vi "Lab Panel V5.25.vi"() -> ()   [LabVIEW 2017] (continued)
                                n852 = Bundle(cluster=w1518, "TL"=w1516, "TN"=w1516) -> (w1517:cluster{"TL":dbl, "TN":dbl})
                                n853 = local write "TEMP START LAB03-2"(w1517) -> ()
                              }
                            }
                          }
                        }
                      }
                    }
                  }
                }
              }
              event "RUN LAB04-1": Value Change {
                n854 = event-data() -> ("NewVal"=w1523:bool)  [unwired: 1 in, 5 out]
                n855 = local write "run lab04-1"(w1523) -> ()
                n856 = case shown="True" w1523 {
                  tunnel: w1529 -> [_ w1567]
                  tunnel: w1528 -> [_ w1566]
                  tunnel: w1526 -> [w1531 w1565]
                  tunnel: w1527 -> [_ w1564]
                  tunnel: w1525 -> [_ w1563]
                  tunnel: [w1530 w1562] -> w1524
                  tunnel: w1522 -> [_ w1561]
                  tunnel: w1521 -> [_ w1560]
                  tunnel: w1520 -> [_ w1559]
                  tunnel: w1519 -> [_ w1557]
                  frame False {
                    # "stop test"
                    n857 = stacked-sequence {
                      tunnel: w1531 -> [w1540 _]
                      tunnel: [w1532 _] -> w1530
                      frame #0 {
                        n858 = local read "DISP LAB04-1"() -> (w1539:T4)
                        n859 = Unbundle(w1539) -> ("CYCLE"=w1537:dbl, "MINS"=w1538:dbl)  [unwired: 1 out]
                        n860 = case shown="\"CYCLE TEST\"" w1540 {
                          tunnel: w1538 -> [_ _ w1547]
                          tunnel: w1537 -> [w1545 w1546 _]
                          tunnel: [w1545 w1546 w1547] -> w1536
                          frame "CHART TEST", Default {
                          }
                          frame "CYCLE TEST" {
                          }
                          frame "T-RISE TEST" {
                          }
                        }
                        n861 = local read "TDMS LAB04-1"() -> (w1544:refnum<k34>)
                        n862 = Build Array("STOPPED") -> (w1541:string[])
                        n863 = Build Array(w1536) -> (w1535:dbl[])
                        n864 = TDMS Write(0:w1544, 5:"TEST RESULT", 7:w1541, 9:w1535) -> (4:w1533:refnum<k34>, 15:w1534:errorcluster)  [unwired: 2 in, 2 out]
                        n865 = TDMS Close(8:w1534, 11:w1533) -> (0:w1532:errorcluster)  [unwired: 1 out]
                      }
                      frame #1 {
                        n866 = local read "DISP LAB04-1"() -> (w1551:T4)
                        n867 = stacked-sequence {
                          tunnel: "LAB04-1" -> [w1553 w1555]
                          frame #0 {
                            n868 = call "sub vi - defrag tdms v1.vi"("panel id"=w1553) -> ("error out"=w1552:errorcluster)  [unwired: 10 in]
                            n869 = local write "data file error"(w1552) -> ()
                          }
                          frame #1 {
                            n870 = call "Save data file (stop) v3.vi"("panel id"=w1555) -> ("network file save error"=w1554:errorcluster)  [unwired: 9 in, 1 out]
                            n871 = local write "RESULT LAB04-1"(FALSE) -> ()
                            n872 = local write "data file error"(w1554) -> ()
                          }
                        }
                        n873 = Bundle(cluster=w1551, "STATUS"="STOP") -> (w1549:T4)  [unwired: 2 in]
                        n874 = local write "DISP LAB04-1"(w1549) -> ()
                      }
                    }
                  }
                  frame True {
                    n875 = local read "SIG LAB04-1"() -> (w1558:T2)
                    n876 = stacked-sequence {
                      seq-local: [w1569 _] -> [_ w1573]
                      tunnel: w1567 -> [_ w1583]
                      tunnel: w1566 -> [_ w1582]
                      tunnel: w1565 -> [_ w1581]
                      tunnel: w1564 -> [_ w1580]
                      tunnel: w1563 -> [_ w1579]
                      tunnel: [_ w1578] -> w1562
                      tunnel: w1561 -> [_ w1577]
                      tunnel: w1560 -> [_ w1576]
                      tunnel: w1559 -> [_ w1575]
                      tunnel: w1558 -> [w1568 w1574]
                      tunnel: w1557 -> [_ w1572]
                      frame #0 {
                        n877 = Unbundle(w1568) -> ("AMPS"=w1571:dbl)  [unwired: 4 out]
                        n878 = call "Check For Amps on v1.vi"("ID"="LAB04-1", "amps"=w1571) -> ("amps"=w1569:bool)  [unwired: 9 in]
                      }
                      frame #1 {
                        n879 = case shown="True" w1573 {
                          tunnel: w1583 -> [_ w1596]
                          tunnel: w1582 -> [_ w1595]
                          tunnel: w1581 -> [_ w1594]
                          tunnel: w1580 -> [_ w1593]
                          tunnel: w1579 -> [_ w1592]
                          tunnel: [errorcluster {"status"=FALSE, "code"=0, "source"=""} ("error out") w1591] -> w1578
                          tunnel: w1577 -> [_ w1590]
                          tunnel: w1576 -> [_ w1589]
                          tunnel: w1575 -> [_ w1588]
                          tunnel: w1574 -> [_ w1587]
                          tunnel: w1572 -> [_ w1586]
                          frame False {
                            w1584 = FALSE
                            n880 = local write "RUN LAB04-1"(w1584) -> ()
                            n881 = local write "run lab04-1"(w1584) -> ()
                          }
                          frame True {
                            n882 = stacked-sequence {
                              seq-local: [w1597 _ _ _ _] -> [_ w1621 _ _ _]
                              tunnel: w1596 -> [w1602 _ _ _ _]
                              tunnel: w1595 -> [w1598 _ _ _ _]
                              tunnel: w1594 -> [w1612 _ _ _ _]
                              tunnel: w1593 -> [w1605 _ _ _ _]
                              tunnel: w1592 -> [w1600 _ _ _ _]
                              tunnel: [_ w1616 _ _ _] -> w1591
                              tunnel: w1590 -> [_ _ _ w1642 _]
                              tunnel: w1589 -> [_ _ _ w1641 _]
                              tunnel: w1588 -> [_ _ _ w1640 _]
                              tunnel: w1587 -> [_ _ _ _ _]
                              tunnel: w1586 -> [_ _ _ _ w1656]
                              frame #0 {
                                w1599 = "\\"
                                n883 = local read "SET LAB04-1"() -> (w1607:T5)
                                n884 = case shown="\"CYCLE TEST\"" w1612 {
                                tunnel: ["L04-1-CHART TEST-" "L04-1-CYCLE TEST-" "L04-1-T-RISE TEST-"] -> w1608
                                frame "CHART TEST", Default {
                                }
                                frame "CYCLE TEST" {
                                }
                                frame "T-RISE TEST" {
                                }
                                }
                                n885 = Unbundle(w1607) -> ("DESCRIPTION"=w1606:string)  [unwired: 4 out]
                                n886 = Concatenate Strings(w1602, "\\", w1600, w1599, w1598, w1599) -> (w1609:string)
                                n887 = String To Path(string=w1609) -> (path=w1611:path)
                                n888 = Concatenate Strings(w1609, w1608, w1606, "-", w1605, ".tdms") -> (w1597:string)
                                n889 = Create Folder(path (use dialog)=w1611) -> (error out=w1610:errorcluster)  [unwired: 2 in, 2 out]
                                n890 = global write "Global 1.vi" "LAB04-1 FILE"(w1597) -> ()
                                n891 = call <vilib>:"Clear Errors.vi"("error in (no error)"=w1610) -> ()  [unwired: 5 in, 2 out]
                              }
                              frame #1 {
                                (unwired) FALSE
                                n892 = String To Path(string=w1621) -> (path=w1617:path)
                                n893 = TDMS Open(6:FALSE, 10:T21."create or replace" ("operation (0:open)"), 11:w1617) -> (0:w1616:errorcluster, 3:→"TDMS LAB04-1":refnum<k34>)  [unwired: 4 in]
                              }
                              frame #2 {
                                n894 = local read "SET LAB04-1"() -> (w1627:T5)
                                n895 = local read "TDMS LAB04-1"() -> (w1638:refnum<k34>)
                                n896 = Build Array("Testers Name", "Description", "Set Test Cycles", "T-Rise minutes", "T-Rise Deg C") -> (w1628:string[])
                                n897 = Unbundle(w1627) -> ("NAME"=w1626:string, "DESCRIPTION"=w1625:string, "CYCLES"=w1624:dbl, "T-RISE mins"=w1623:dbl, "T-RISE deg C"=w1622:dbl)
                                n898 = Number To Decimal String(number=w1624) -> (decimal integer string=w1637:string)  [unwired: 1 in]
                                n899 = Number To Decimal String(number=w1623) -> (decimal integer string=w1636:string)  [unwired: 1 in]
                                n900 = Number To Decimal String(number=w1622) -> (decimal integer string=w1635:string)  [unwired: 1 in]
                                n901 = Build Array(w1626, w1625, w1637, w1636, w1635) -> (w1634:string[])
                                n902 = TDMS Set Properties(5:w1634, 7:w1628, 11:w1638) -> ()  [unwired: 3 in, 4 out]
                              }
                              frame #3 {
                                n903 = local read "DISP LAB04-1"() -> (w1643:T4)
                                n904 = Concatenate Strings("LAB04-1  ", w1642) -> (w1644:string)
                                n905 = Two Button Dialog(message=w1644, 1:w1640, 2:w1641) -> (T button?=w1646:bool)
                                n906 = case shown="True" w1646 {
                                tunnel: w1643 -> [w1653 w1654]
                                tunnel: [w1653 w1654] -> w1650
                                tunnel: [w1652 w1655] -> w1649
                                tunnel: [w1651 w1655] -> w1648
                                frame False {
                                n907 = Unbundle(w1653) -> ("CYCLE"=w1652:dbl, "MINS"=w1651:dbl)  [unwired: 1 out]
                                }
                                frame True {
                                w1655 = 0.0
                                }
                                }
                                n908 = Bundle(cluster=w1650, "CYCLE"=w1649, "MINS"=w1648, "STATUS"="RUN") -> (w1639:T4)
                                n909 = local write "DISP LAB04-1"(w1639) -> ()
                              }
                              frame #4 {
                                n910 = local read "TEMP START LAB04-1"() -> (w1658:cluster{"TL":dbl, "TN":dbl})
                                n911 = Bundle(cluster=w1658, "TL"=w1656, "TN"=w1656) -> (w1657:cluster{"TL":dbl, "TN":dbl})
                                n912 = local write "TEMP START LAB04-1"(w1657) -> ()
                              }
                            }
                          }
                        }
                      }
                    }
                  }
                }
              }
              event "RUN LAB04-2": Value Change {
                n913 = event-data() -> ("NewVal"=w1663:bool)  [unwired: 1 in, 5 out]
                n914 = local write "run lab04-2"(w1663) -> ()
                n915 = case shown="True" w1663 {
                  tunnel: w1669 -> [_ w1707]
                  tunnel: w1668 -> [_ w1706]
                  tunnel: w1666 -> [w1671 w1705]
                  tunnel: w1667 -> [_ w1704]
                  tunnel: w1665 -> [_ w1703]
                  tunnel: [w1670 w1702] -> w1664
                  tunnel: w1662 -> [_ w1701]
                  tunnel: w1661 -> [_ w1700]
                  tunnel: w1660 -> [_ w1699]
                  tunnel: w1659 -> [_ w1697]
                  frame False {
                    # "stop test"
                    n916 = stacked-sequence {
                      tunnel: w1671 -> [w1680 _]
                      tunnel: [w1672 _] -> w1670
                      frame #0 {
                        n917 = local read "DISP LAB04-2"() -> (w1679:T4)
                        n918 = Unbundle(w1679) -> ("CYCLE"=w1677:dbl, "MINS"=w1678:dbl)  [unwired: 1 out]
                        n919 = case shown="\"CYCLE TEST\"" w1680 {
                          tunnel: w1678 -> [_ _ w1687]
                          tunnel: w1677 -> [w1685 w1686 _]
                          tunnel: [w1685 w1686 w1687] -> w1676
                          frame "CHART TEST", Default {
                          }
                          frame "CYCLE TEST" {
                          }
                          frame "T-RISE TEST" {
                          }
                        }
                        n920 = local read "TDMS LAB04-2"() -> (w1684:refnum<k34>)
                        n921 = Build Array("STOPPED") -> (w1681:string[])
                        n922 = Build Array(w1676) -> (w1675:dbl[])
                        n923 = TDMS Write(0:w1684, 5:"TEST RESULT", 7:w1681, 9:w1675) -> (4:w1673:refnum<k34>, 15:w1674:errorcluster)  [unwired: 2 in, 2 out]
                        n924 = TDMS Close(8:w1674, 11:w1673) -> (0:w1672:errorcluster)  [unwired: 1 out]
                      }
                      frame #1 {
                        n925 = local read "DISP LAB04-2"() -> (w1691:T4)
                        n926 = stacked-sequence {
                          tunnel: "LAB04-2" -> [w1693 w1695]
                          frame #0 {
                            n927 = call "sub vi - defrag tdms v1.vi"("panel id"=w1693) -> ("error out"=w1692:errorcluster)  [unwired: 10 in]
                            n928 = local write "data file error"(w1692) -> ()
                          }
                          frame #1 {
                            n929 = call "Save data file (stop) v3.vi"("panel id"=w1695) -> ("network file save error"=w1694:errorcluster)  [unwired: 9 in, 1 out]
                            n930 = local write "RESULT LAB04-2"(FALSE) -> ()
                            n931 = local write "data file error"(w1694) -> ()
                          }
                        }
                        n932 = Bundle(cluster=w1691, "STATUS"="STOP") -> (w1689:T4)  [unwired: 2 in]
                        n933 = local write "DISP LAB04-2"(w1689) -> ()
                      }
                    }
                  }
                  frame True {
                    n934 = local read "SIG LAB04-2"() -> (w1698:T2)
                    n935 = stacked-sequence {
                      seq-local: [w1709 _] -> [_ w1713]
                      tunnel: w1707 -> [_ w1723]
                      tunnel: w1706 -> [_ w1722]
                      tunnel: w1705 -> [_ w1721]
                      tunnel: w1704 -> [_ w1720]
                      tunnel: w1703 -> [_ w1719]
                      tunnel: [_ w1718] -> w1702
                      tunnel: w1701 -> [_ w1717]
                      tunnel: w1700 -> [_ w1716]
                      tunnel: w1699 -> [_ w1715]
                      tunnel: w1698 -> [w1708 w1714]
                      tunnel: w1697 -> [_ w1712]
                      frame #0 {
                        n936 = Unbundle(w1708) -> ("AMPS"=w1711:dbl)  [unwired: 4 out]
                        n937 = call "Check For Amps on v1.vi"("ID"="LAB04-2", "amps"=w1711) -> ("amps"=w1709:bool)  [unwired: 9 in]
                      }
                      frame #1 {
                        n938 = case shown="True" w1713 {
                          tunnel: w1723 -> [_ w1736]
                          tunnel: w1722 -> [_ w1735]
                          tunnel: w1721 -> [_ w1734]
                          tunnel: w1720 -> [_ w1733]
                          tunnel: w1719 -> [_ w1732]
                          tunnel: [errorcluster {"status"=FALSE, "code"=0, "source"=""} ("error out") w1731] -> w1718
                          tunnel: w1717 -> [_ w1730]
                          tunnel: w1716 -> [_ w1729]
                          tunnel: w1715 -> [_ w1728]
                          tunnel: w1714 -> [_ w1727]
                          tunnel: w1712 -> [_ w1726]
                          frame False {
                            w1724 = FALSE
                            n939 = local write "RUN LAB04-2"(w1724) -> ()
                            n940 = local write "run lab04-2"(w1724) -> ()
                          }
                          frame True {
                            n941 = stacked-sequence {
                              seq-local: [w1737 _ _ _ _] -> [_ w1761 _ _ _]
                              tunnel: w1736 -> [w1742 _ _ _ _]
                              tunnel: w1735 -> [w1738 _ _ _ _]
                              tunnel: w1734 -> [w1752 _ _ _ _]
                              tunnel: w1733 -> [w1745 _ _ _ _]
                              tunnel: w1732 -> [w1740 _ _ _ _]
                              tunnel: [_ w1756 _ _ _] -> w1731
                              tunnel: w1730 -> [_ _ _ w1782 _]
                              tunnel: w1729 -> [_ _ _ w1781 _]
                              tunnel: w1728 -> [_ _ _ w1780 _]
                              tunnel: w1727 -> [_ _ _ _ _]
                              tunnel: w1726 -> [_ _ _ _ w1796]
                              frame #0 {
                                w1739 = "\\"
                                n942 = local read "SET LAB04-2"() -> (w1747:T5)
                                n943 = case shown="\"CHART TEST\", Default" w1752 {
                                tunnel: ["L04-2-CHART TEST-" "L04-2-CYCLE TEST-" "L04-2-T-RISE TEST-"] -> w1748
                                frame "CHART TEST", Default {
                                }
                                frame "CYCLE TEST" {
                                }
                                frame "T-RISE TEST" {
                                }
                                }
                                n944 = Unbundle(w1747) -> ("DESCRIPTION"=w1746:string)  [unwired: 4 out]
                                n945 = Concatenate Strings(w1742, "\\", w1740, w1739, w1738, w1739) -> (w1749:string)
                                n946 = String To Path(string=w1749) -> (path=w1751:path)
                                n947 = Concatenate Strings(w1749, w1748, w1746, "-", w1745, ".tdms") -> (w1737:string)
                                n948 = Create Folder(path (use dialog)=w1751) -> (error out=w1750:errorcluster)  [unwired: 2 in, 2 out]
                                n949 = global write "Global 1.vi" "LAB04-2 FILE"(w1737) -> ()
                                n950 = call <vilib>:"Clear Errors.vi"("error in (no error)"=w1750) -> ()  [unwired: 5 in, 2 out]
                              }
                              frame #1 {
                                (unwired) FALSE
                                n951 = String To Path(string=w1761) -> (path=w1757:path)
                                n952 = TDMS Open(6:FALSE, 10:T21."create or replace" ("operation (0:open)"), 11:w1757) -> (0:w1756:errorcluster, 3:→"TDMS LAB04-2":refnum<k34>)  [unwired: 4 in]
                              }
                              frame #2 {
                                n953 = local read "SET LAB04-2"() -> (w1767:T5)
                                n954 = local read "TDMS LAB04-2"() -> (w1778:refnum<k34>)
                                n955 = Build Array("Testers Name", "Description", "Set Test Cycles", "T-Rise minutes", "T-Rise Deg C") -> (w1768:string[])
                                n956 = Unbundle(w1767) -> ("NAME"=w1766:string, "DESCRIPTION"=w1765:string, "CYCLES"=w1764:dbl, "T-RISE mins"=w1763:dbl, "T-RISE deg C"=w1762:dbl)
                                n957 = Number To Decimal String(number=w1764) -> (decimal integer string=w1777:string)  [unwired: 1 in]
                                n958 = Number To Decimal String(number=w1763) -> (decimal integer string=w1776:string)  [unwired: 1 in]
                                n959 = Number To Decimal String(number=w1762) -> (decimal integer string=w1775:string)  [unwired: 1 in]
                                n960 = Build Array(w1766, w1765, w1777, w1776, w1775) -> (w1774:string[])
                                n961 = TDMS Set Properties(5:w1774, 7:w1768, 11:w1778) -> ()  [unwired: 3 in, 4 out]
                              }
                              frame #3 {
                                n962 = local read "DISP LAB04-2"() -> (w1783:T4)
                                n963 = Concatenate Strings("LAB04-2 ", w1782) -> (w1784:string)
                                n964 = Two Button Dialog(message=w1784, 1:w1780, 2:w1781) -> (T button?=w1786:bool)
                                n965 = case shown="True" w1786 {
                                tunnel: w1783 -> [w1793 w1794]
                                tunnel: [w1793 w1794] -> w1790
                                tunnel: [w1792 w1795] -> w1789
                                tunnel: [w1791 w1795] -> w1788
                                frame False {
                                n966 = Unbundle(w1793) -> ("CYCLE"=w1792:dbl, "MINS"=w1791:dbl)  [unwired: 1 out]
                                }
                                frame True {
                                w1795 = 0.0
                                }
                                }
                                n967 = Bundle(cluster=w1790, "CYCLE"=w1789, "MINS"=w1788, "STATUS"="RUN") -> (w1779:T4)
                                n968 = local write "DISP LAB04-2"(w1779) -> ()
                              }
                              frame #4 {
                                n969 = local read "TEMP START LAB04-2"() -> (w1798:cluster{"TL":dbl, "TN":dbl})
                                n970 = Bundle(cluster=w1798, "TL"=w1796, "TN"=w1796) -> (w1797:cluster{"TL":dbl, "TN":dbl})
                                n971 = local write "TEMP START LAB04-2"(w1797) -> ()
                              }
                            }
                          }
                        }
                      }
                    }
                  }
                }
              }
              event "RUN LAB05-1": Value Change {
                n972 = event-data() -> ("NewVal"=w1803:bool)  [unwired: 1 in, 5 out]
                n973 = local write "run lab05-1"(w1803) -> ()
                n974 = case shown="True" w1803 {
                  tunnel: w1809 -> [_ w1847]
                  tunnel: w1808 -> [_ w1846]
                  tunnel: w1806 -> [w1811 w1845]
                  tunnel: w1807 -> [_ w1844]
                  tunnel: w1805 -> [_ w1843]
                  tunnel: [w1810 w1842] -> w1804
                  tunnel: w1802 -> [_ w1841]
                  tunnel: w1801 -> [_ w1840]
                  tunnel: w1800 -> [_ w1839]
                  tunnel: w1799 -> [_ w1837]
                  frame False {
                    # "stop test"
                    n975 = stacked-sequence {
                      tunnel: w1811 -> [w1820 _]
                      tunnel: [w1812 _] -> w1810
                      frame #0 {
                        n976 = local read "DISP LAB05-1"() -> (w1819:T4)
                        n977 = Unbundle(w1819) -> ("CYCLE"=w1817:dbl, "MINS"=w1818:dbl)  [unwired: 1 out]
                        n978 = case shown="\"CYCLE TEST\"" w1820 {
                          tunnel: w1818 -> [_ _ w1827]
                          tunnel: w1817 -> [w1825 w1826 _]
                          tunnel: [w1825 w1826 w1827] -> w1816
                          frame "CHART TEST", Default {
                          }
                          frame "CYCLE TEST" {
                          }
                          frame "T-RISE TEST" {
                          }
                        }
                        n979 = local read "TDMS LAB05-1"() -> (w1824:refnum<k34>)
                        n980 = Build Array("STOPPED") -> (w1821:string[])
                        n981 = Build Array(w1816) -> (w1815:dbl[])
                        n982 = TDMS Write(0:w1824, 5:"TEST RESULT", 7:w1821, 9:w1815) -> (4:w1813:refnum<k34>, 15:w1814:errorcluster)  [unwired: 2 in, 2 out]
                        n983 = TDMS Close(8:w1814, 11:w1813) -> (0:w1812:errorcluster)  [unwired: 1 out]
                      }
                      frame #1 {
                        n984 = local read "DISP LAB05-1"() -> (w1831:T4)
                        n985 = stacked-sequence {
                          tunnel: "LAB05-1" -> [w1833 w1835]
                          frame #0 {
                            n986 = call "sub vi - defrag tdms v1.vi"("panel id"=w1833) -> ("error out"=w1832:errorcluster)  [unwired: 10 in]
                            n987 = local write "data file error"(w1832) -> ()
                          }
                          frame #1 {
                            n988 = call "Save data file (stop) v3.vi"("panel id"=w1835) -> ("network file save error"=w1834:errorcluster)  [unwired: 9 in, 1 out]
                            n989 = local write "RESULT LAB05-1"(FALSE) -> ()
                            n990 = local write "data file error"(w1834) -> ()
                          }
                        }
                        n991 = Bundle(cluster=w1831, "STATUS"="STOP") -> (w1829:T4)  [unwired: 2 in]
                        n992 = local write "DISP LAB05-1"(w1829) -> ()
                      }
                    }
                  }
                  frame True {
                    n993 = local read "SIG LAB05-1"() -> (w1838:T2)
                    n994 = stacked-sequence {
                      seq-local: [w1849 _] -> [_ w1853]
                      tunnel: w1847 -> [_ w1863]
                      tunnel: w1846 -> [_ w1862]
                      tunnel: w1845 -> [_ w1861]
                      tunnel: w1844 -> [_ w1860]
                      tunnel: w1843 -> [_ w1859]
                      tunnel: [_ w1858] -> w1842
                      tunnel: w1841 -> [_ w1857]
                      tunnel: w1840 -> [_ w1856]
                      tunnel: w1839 -> [_ w1855]
                      tunnel: w1838 -> [w1848 w1854]
                      tunnel: w1837 -> [_ w1852]
                      frame #0 {
                        n995 = Unbundle(w1848) -> ("AMPS"=w1851:dbl)  [unwired: 4 out]
                        n996 = call "Check For Amps on v1.vi"("ID"="LAB05-1", "amps"=w1851) -> ("amps"=w1849:bool)  [unwired: 9 in]
                      }
                      frame #1 {
                        n997 = case shown="True" w1853 {
                          tunnel: w1863 -> [_ w1876]
                          tunnel: w1862 -> [_ w1875]
                          tunnel: w1861 -> [_ w1874]
                          tunnel: w1860 -> [_ w1873]
                          tunnel: w1859 -> [_ w1872]
                          tunnel: [errorcluster {"status"=FALSE, "code"=0, "source"=""} ("error out") w1871] -> w1858
                          tunnel: w1857 -> [_ w1870]
                          tunnel: w1856 -> [_ w1869]
                          tunnel: w1855 -> [_ w1868]
                          tunnel: w1854 -> [_ w1867]
                          tunnel: w1852 -> [_ w1866]
                          frame False {
                            w1864 = FALSE
                            n998 = local write "RUN LAB05-1"(w1864) -> ()
                            n999 = local write "run lab05-1"(w1864) -> ()
                          }
                          frame True {
                            n1000 = stacked-sequence {
                              seq-local: [w1877 _ _ _ _] -> [_ w1901 _ _ _]
                              tunnel: w1876 -> [w1882 _ _ _ _]
                              tunnel: w1875 -> [w1878 _ _ _ _]
                              tunnel: w1874 -> [w1892 _ _ _ _]
                              tunnel: w1873 -> [w1885 _ _ _ _]
                              tunnel: w1872 -> [w1880 _ _ _ _]
                              tunnel: [_ w1896 _ _ _] -> w1871
                              tunnel: w1870 -> [_ _ _ w1921 _]
                              tunnel: w1869 -> [_ _ _ w1920 _]
                              tunnel: w1868 -> [_ _ _ w1919 _]
                              tunnel: w1867 -> [_ _ _ _ _]
                              tunnel: w1866 -> [_ _ _ _ w1936]
                              frame #0 {
                                w1879 = "\\"
                                n1001 = local read "SET LAB05-1"() -> (w1887:T5)
                                n1002 = case shown="\"CYCLE TEST\"" w1892 {
                                tunnel: ["L05-1-CHART TEST-" "L05-1-CYCLE TEST-" "L05-1-T-RISE TEST-"] -> w1888
                                frame "CHART TEST", Default {
                                }
                                frame "CYCLE TEST" {
                                }
                                frame "T-RISE TEST" {
                                }
                                }
                                n1003 = Unbundle(w1887) -> ("DESCRIPTION"=w1886:string)  [unwired: 4 out]
                                n1004 = Concatenate Strings(w1882, "\\", w1880, w1879, w1878, w1879) -> (w1889:string)
                                n1005 = String To Path(string=w1889) -> (path=w1891:path)
                                n1006 = Concatenate Strings(w1889, w1888, w1886, "-", w1885, ".tdms") -> (w1877:string)
                                n1007 = Create Folder(path (use dialog)=w1891) -> (error out=w1890:errorcluster)  [unwired: 2 in, 2 out]
                                n1008 = global write "Global 1.vi" "LAB05-1 FILE"(w1877) -> ()
                                n1009 = call <vilib>:"Clear Errors.vi"("error in (no error)"=w1890) -> ()  [unwired: 5 in, 2 out]
                              }
                              frame #1 {
                                (unwired) FALSE
                                n1010 = String To Path(string=w1901) -> (path=w1897:path)
                                n1011 = TDMS Open(6:FALSE, 10:T21."create or replace" ("operation (0:open)"), 11:w1897) -> (0:w1896:errorcluster, 3:→"TDMS LAB05-1":refnum<k34>)  [unwired: 4 in]
                              }
                              frame #2 {
                                n1012 = local read "SET LAB05-1"() -> (w1907:T5)
                                n1013 = local read "TDMS LAB05-1"() -> (w1918:refnum<k34>)
                                n1014 = Build Array("Testers Name", "Description", "Set Test Cycles", "T-Rise minutes", "T-Rise Deg C") -> (w1908:string[])
                                n1015 = Unbundle(w1907) -> ("NAME"=w1906:string, "DESCRIPTION"=w1905:string, "CYCLES"=w1904:dbl, "T-RISE mins"=w1903:dbl, "T-RISE deg C"=w1902:dbl)
                                n1016 = Number To Decimal String(number=w1904) -> (decimal integer string=w1917:string)  [unwired: 1 in]
                                n1017 = Number To Decimal String(number=w1903) -> (decimal integer string=w1916:string)  [unwired: 1 in]
                                n1018 = Number To Decimal String(number=w1902) -> (decimal integer string=w1915:string)  [unwired: 1 in]
                                n1019 = Build Array(w1906, w1905, w1917, w1916, w1915) -> (w1914:string[])
                                n1020 = TDMS Set Properties(5:w1914, 7:w1908, 11:w1918) -> ()  [unwired: 3 in, 4 out]
                              }
                              frame #3 {
                                n1021 = local read "DISP LAB05-1"() -> (w1923:T4)
                                n1022 = Concatenate Strings("LAB05-1  ", w1921) -> (w1924:string)
                                n1023 = Two Button Dialog(message=w1924, 1:w1919, 2:w1920) -> (T button?=w1926:bool)
                                n1024 = case shown="True" w1926 {
                                tunnel: w1923 -> [w1933 w1934]
                                tunnel: [w1933 w1934] -> w1930
                                tunnel: [w1932 w1935] -> w1929
                                tunnel: [w1931 w1935] -> w1928
                                frame False {
                                n1025 = Unbundle(w1933) -> ("CYCLE"=w1932:dbl, "MINS"=w1931:dbl)  [unwired: 1 out]
                                }
                                frame True {
                                w1935 = 0.0
                                }
                                }
                                n1026 = Bundle(cluster=w1930, "CYCLE"=w1929, "MINS"=w1928, "STATUS"="RUN") -> (w1922:T4)
                                n1027 = local write "DISP LAB05-1"(w1922) -> ()
                              }
                              frame #4 {
                                n1028 = local read "TEMP START LAB05-1"() -> (w1938:cluster{"TL":dbl, "TN":dbl})
                                n1029 = Bundle(cluster=w1938, "TL"=w1936, "TN"=w1936) -> (w1937:cluster{"TL":dbl, "TN":dbl})
                                n1030 = local write "TEMP START LAB05-1"(w1937) -> ()
                              }
                            }
                          }
                        }
                      }
                    }
                  }
                }
              }
              event "RUN LAB05-2": Value Change {
                n1031 = event-data() -> ("NewVal"=w1944:bool)  [unwired: 1 in, 5 out]
                n1032 = local read "SIG LAB05-2"() -> (w1940:T2)
                n1033 = case shown="True" w1944 {
                  tunnel: w1950 -> [_ w1988]
                  tunnel: w1949 -> [_ w1987]
                  tunnel: w1947 -> [w1952 w1986]
                  tunnel: w1948 -> [_ w1985]
                  tunnel: w1946 -> [_ w1984]
                  tunnel: [w1951 w1983] -> w1945
                  tunnel: w1943 -> [_ w1982]
                  tunnel: w1942 -> [_ w1981]
                  tunnel: w1941 -> [_ w1980]
                  tunnel: w1940 -> [_ w1979]
                  tunnel: w1939 -> [_ w1978]
                  frame False {
                    # "stop test"
                    n1034 = stacked-sequence {
                      tunnel: w1952 -> [w1961 _]
                      tunnel: [w1953 _] -> w1951
                      frame #0 {
                        n1035 = local read "DISP LAB05-2"() -> (w1960:T4)
                        n1036 = Unbundle(w1960) -> ("CYCLE"=w1958:dbl, "MINS"=w1959:dbl)  [unwired: 1 out]
                        n1037 = case shown="\"CYCLE TEST\"" w1961 {
                          tunnel: w1959 -> [_ _ w1968]
                          tunnel: w1958 -> [w1966 w1967 _]
                          tunnel: [w1966 w1967 w1968] -> w1957
                          frame "CHART TEST", Default {
                          }
                          frame "CYCLE TEST" {
                          }
                          frame "T-RISE TEST" {
                          }
                        }
                        n1038 = local read "TDMS LAB05-2"() -> (w1965:refnum<k34>)
                        n1039 = Build Array("STOPPED") -> (w1962:string[])
                        n1040 = Build Array(w1957) -> (w1956:dbl[])
                        n1041 = TDMS Write(0:w1965, 5:"TEST RESULT", 7:w1962, 9:w1956) -> (4:w1954:refnum<k34>, 15:w1955:errorcluster)  [unwired: 2 in, 2 out]
                        n1042 = TDMS Close(8:w1955, 11:w1954) -> (0:w1953:errorcluster)  [unwired: 1 out]
                      }
                      frame #1 {
                        n1043 = local read "DISP LAB05-2"() -> (w1972:T4)
                        n1044 = stacked-sequence {
                          tunnel: "LAB05-2" -> [w1974 w1976]
                          frame #0 {
                            n1045 = call "sub vi - defrag tdms v1.vi"("panel id"=w1974) -> ("error out"=w1973:errorcluster)  [unwired: 10 in]
                            n1046 = local write "data file error"(w1973) -> ()
                          }
                          frame #1 {
                            n1047 = local write "RESULT LAB05-2"(FALSE) -> ()
                            n1048 = call "Save data file (stop) v3.vi"("panel id"=w1976) -> ("network file save error"=w1975:errorcluster)  [unwired: 9 in, 1 out]
                            n1049 = local write "data file error"(w1975) -> ()
                          }
                        }
                        n1050 = Bundle(cluster=w1972, "STATUS"="STOP") -> (w1970:T4)  [unwired: 2 in]
                        n1051 = local write "DISP LAB05-2"(w1970) -> ()
                      }
                    }
                  }
                  frame True {
                    n1052 = stacked-sequence {
                      seq-local: [w1990 _] -> [_ w1994]
                      tunnel: w1988 -> [_ w2004]
                      tunnel: w1987 -> [_ w2003]
                      tunnel: w1986 -> [_ w2002]
                      tunnel: w1985 -> [_ w2001]
                      tunnel: w1984 -> [_ w2000]
                      tunnel: [_ w1999] -> w1983
                      tunnel: w1982 -> [_ w1998]
                      tunnel: w1981 -> [_ w1997]
                      tunnel: w1980 -> [_ w1996]
                      tunnel: w1979 -> [w1989 w1995]
                      tunnel: w1978 -> [_ w1993]
                      frame #0 {
                        n1053 = Unbundle(w1989) -> ("AMPS"=w1992:dbl)  [unwired: 4 out]
                        n1054 = call "Check For Amps on v1.vi"("ID"="LAB05-2", "amps"=w1992) -> ("amps"=w1990:bool)  [unwired: 9 in]
                      }
                      frame #1 {
                        n1055 = case shown="True" w1994 {
                          tunnel: w2004 -> [_ w2017]
                          tunnel: w2003 -> [_ w2016]
                          tunnel: w2002 -> [_ w2015]
                          tunnel: w2001 -> [_ w2014]
                          tunnel: w2000 -> [_ w2013]
                          tunnel: [errorcluster {"status"=FALSE, "code"=0, "source"=""} ("error out") w2012] -> w1999
                          tunnel: w1998 -> [_ w2011]
                          tunnel: w1997 -> [_ w2010]
                          tunnel: w1996 -> [_ w2009]
                          tunnel: w1995 -> [_ w2008]
                          tunnel: w1993 -> [_ w2007]
                          frame False {
                            w2005 = FALSE
                            n1056 = local write "RUN LAB05-2"(w2005) -> ()
                            n1057 = local write "run lab05-2"(w2005) -> ()
                          }
                          frame True {
                            n1058 = stacked-sequence {
                              seq-local: [w2018 _ _ _ _] -> [_ w2042 _ _ _]
                              tunnel: w2017 -> [w2023 _ _ _ _]
                              tunnel: w2016 -> [w2019 _ _ _ _]
                              tunnel: w2015 -> [w2033 _ _ _ _]
                              tunnel: w2014 -> [w2026 _ _ _ _]
                              tunnel: w2013 -> [w2021 _ _ _ _]
                              tunnel: [_ w2037 _ _ _] -> w2012
                              tunnel: w2011 -> [_ _ _ w2062 _]
                              tunnel: w2010 -> [_ _ _ w2061 _]
                              tunnel: w2009 -> [_ _ _ w2060 _]
                              tunnel: w2008 -> [_ _ _ _ _]
                              tunnel: w2007 -> [_ _ _ _ w2077]
                              frame #0 {
                                w2020 = "\\"
                                n1059 = local read "SET LAB05-2"() -> (w2028:T5)
                                n1060 = case shown="\"CYCLE TEST\"" w2033 {
                                tunnel: ["L05-2-CHART TEST-" "L05-2-CYCLE TEST-" "L05-2-T-RISE TEST-"] -> w2029
                                frame "CHART TEST", Default {
                                }
                                frame "CYCLE TEST" {
                                }
                                frame "T-RISE TEST" {
                                }
                                }
                                n1061 = Unbundle(w2028) -> ("DESCRIPTION"=w2027:string)  [unwired: 4 out]
                                n1062 = Concatenate Strings(w2023, "\\", w2021, w2020, w2019, w2020) -> (w2030:string)
                                n1063 = String To Path(string=w2030) -> (path=w2032:path)
                                n1064 = Concatenate Strings(w2030, w2029, w2027, "-", w2026, ".tdms") -> (w2018:string)
                                n1065 = Create Folder(path (use dialog)=w2032) -> (error out=w2031:errorcluster)  [unwired: 2 in, 2 out]
                                n1066 = global write "Global 1.vi" "LAB05-2 FILE"(w2018) -> ()
                                n1067 = call <vilib>:"Clear Errors.vi"("error in (no error)"=w2031) -> ()  [unwired: 5 in, 2 out]
                              }
                              frame #1 {
                                (unwired) FALSE
                                n1068 = String To Path(string=w2042) -> (path=w2038:path)
                                n1069 = TDMS Open(6:FALSE, 10:T21."create or replace" ("operation (0:open)"), 11:w2038) -> (0:w2037:errorcluster, 3:→"TDMS LAB05-2":refnum<k34>)  [unwired: 4 in]
                              }
                              frame #2 {
                                n1070 = local read "SET LAB05-2"() -> (w2048:T5)
                                n1071 = local read "TDMS LAB05-2"() -> (w2059:refnum<k34>)
                                n1072 = Build Array("Testers Name", "Description", "Set Test Cycles", "T-Rise minutes", "T-Rise Deg C") -> (w2049:string[])
                                n1073 = Unbundle(w2048) -> ("NAME"=w2047:string, "DESCRIPTION"=w2046:string, "CYCLES"=w2045:dbl, "T-RISE mins"=w2044:dbl, "T-RISE deg C"=w2043:dbl)
                                n1074 = Number To Decimal String(number=w2045) -> (decimal integer string=w2058:string)  [unwired: 1 in]
                                n1075 = Number To Decimal String(number=w2044) -> (decimal integer string=w2057:string)  [unwired: 1 in]
                                n1076 = Number To Decimal String(number=w2043) -> (decimal integer string=w2056:string)  [unwired: 1 in]
                                n1077 = Build Array(w2047, w2046, w2058, w2057, w2056) -> (w2055:string[])
                                n1078 = TDMS Set Properties(5:w2055, 7:w2049, 11:w2059) -> ()  [unwired: 3 in, 4 out]
                              }
                              frame #3 {
                                n1079 = local read "DISP LAB05-2"() -> (w2064:T4)
                                n1080 = Concatenate Strings("LAB05-2  ", w2062) -> (w2065:string)
                                n1081 = Two Button Dialog(message=w2065, 1:w2060, 2:w2061) -> (T button?=w2067:bool)
                                n1082 = case shown="True" w2067 {
                                tunnel: w2064 -> [w2074 w2075]
                                tunnel: [w2074 w2075] -> w2071
                                tunnel: [w2073 w2076] -> w2070
                                tunnel: [w2072 w2076] -> w2069
                                frame False {
                                n1083 = Unbundle(w2074) -> ("CYCLE"=w2073:dbl, "MINS"=w2072:dbl)  [unwired: 1 out]
                                }
                                frame True {
                                w2076 = 0.0
                                }
                                }
                                n1084 = Bundle(cluster=w2071, "CYCLE"=w2070, "MINS"=w2069, "STATUS"="RUN") -> (w2063:T4)
                                n1085 = local write "DISP LAB05-2"(w2063) -> ()
                              }
                              frame #4 {
                                n1086 = local read "TEMP START LAB05-2"() -> (w2079:cluster{"TL":dbl, "TN":dbl})
                                n1087 = Bundle(cluster=w2079, "TL"=w2077, "TN"=w2077) -> (w2078:cluster{"TL":dbl, "TN":dbl})
                                n1088 = local write "TEMP START LAB05-2"(w2078) -> ()
                              }
                            }
                          }
                        }
                      }
                    }
                  }
                }
                n1089 = local write "run lab05-2"(w1944) -> ()
              }
            }
            n1090 = local write "data file error"(w648) -> ()
          }
          frame #4 {
            # "check if test cycles reached for cycle tests, if so then test pass"
            n1091 = stacked-sequence {
              tunnel: w2099 -> [_ _ _ _ _ _ _ _ _ _]
              tunnel: w2098 -> [_ _ _ _ _ _ _ _ _ _]
              tunnel: w2097 -> [_ _ _ _ _ _ _ _ _ _]
              tunnel: w2096 -> [_ _ _ _ _ _ _ _ _ _]
              tunnel: w2095 -> [_ _ _ _ _ _ _ _ _ _]
              tunnel: w2094 -> [_ _ _ _ _ _ _ _ _ _]
              tunnel: w2093 -> [_ _ _ _ _ _ _ _ _ _]
              tunnel: w2092 -> [_ _ _ _ _ _ _ _ _ _]
              tunnel: w2091 -> [_ _ _ _ _ _ _ _ _ _]
              tunnel: w2090 -> [_ _ _ _ _ _ _ _ _ _]
              tunnel: w2089 -> [w2105 _ _ _ _ _ _ _ _ _]
              tunnel: w2088 -> [_ w2140 _ _ _ _ _ _ _ _]
              tunnel: w2087 -> [_ _ w2180 _ _ _ _ _ _ _]
              tunnel: w2086 -> [_ _ _ w2220 _ _ _ _ _ _]
              tunnel: w2085 -> [_ _ _ _ w2260 _ _ _ _ _]
              tunnel: w2084 -> [_ _ _ _ _ w2300 _ _ _ _]
              tunnel: w2083 -> [_ _ _ _ _ _ w2340 _ _ _]
              tunnel: w2082 -> [_ _ _ _ _ _ _ w2380 _ _]
              tunnel: w2081 -> [_ _ _ _ _ _ _ _ w2420 _]
              tunnel: w2080 -> [_ _ _ _ _ _ _ _ _ w2460]
              frame #0 {
                # "LAB01-1"
                n1092 = Less?(x=w2105, y=2) -> (x < y?=w2103:bool)
                n1093 = local read "DISP LAB01-1"() -> (w2106:T4)
                n1094 = Unbundle(w2106) -> ("STATUS"=w2100:string)  [unwired: 2 out]
                n1095 = Equal?(x=w2100, y="RUN") -> (x = y?=w2102:bool)
                n1096 = And(x=w2102, y=w2103) -> (x .and. y?=w2101:bool)
                n1097 = case shown="True" w2101 {
                  tunnel: w2106 -> [_ w2111]
                  tunnel: w2105 -> [_ w2115]
                  frame False {
                  }
                  frame True {
                    n1098 = local read "SET LAB01-1"() -> (w2117:T5)
                    n1099 = local read "TDMS LAB01-1"() -> (w2110:refnum<k34>)
                    n1100 = Unbundle(w2117) -> ("CYCLES"=w2108:dbl, "T-RISE mins"=w2114:dbl)  [unwired: 3 out]
                    n1101 = case shown="\"CYCLE TEST\"" w2115 {
                      tunnel: w2114 -> [_ _ w2124]
                      tunnel: [w2119 w2121 w2124] -> w2113
                      tunnel: w2108 -> [w2119 w2121 _]
                      tunnel: ["CHART PASS" "CYCLE PASS" "T-RISE PASS"] -> w2112
                      frame "CHART TEST", Default {
                      }
                      frame "CYCLE TEST" {
                      }
                      frame "T-RISE TEST" {
                      }
                    }
                    n1102 = Unbundle(w2111) -> ("CYCLE"=w2116:dbl)  [unwired: 2 out]
                    n1103 = Increment(x=w2108) -> (x+1=w2109:dbl)
                    n1104 = Greater Or Equal?(x=w2116, y=w2109) -> (x >= y?=w2118:bool)
                    n1105 = case shown="True" w2118 {
                      tunnel: w2113 -> [w2128 _]
                      tunnel: w2112 -> [w2127 _]
                      tunnel: w2111 -> [w2126 _]
                      tunnel: w2110 -> [w2125 _]
                      frame True {
                        n1106 = stacked-sequence {
                          tunnel: w2128 -> [w2132 _]
                          tunnel: w2127 -> [w2130 w2136]
                          tunnel: w2126 -> [_ w2139]
                          tunnel: w2125 -> [w2129 _]
                          frame #0 {
                            n1107 = Build Array(w2130) -> (w2133:string[])
                            n1108 = Build Array(w2132) -> (w2131:dbl[])
                            n1109 = TDMS Write(0:w2129, 5:"TEST PASS", 7:w2133, 9:w2131) -> (15:w2135:errorcluster)  [unwired: 2 in, 3 out]
                            n1110 = local write "data file error"(w2135) -> ()
                          }
                          frame #1 {
                            n1111 = Bundle(cluster=w2139, "STATUS"=w2136) -> (w2137:T4)  [unwired: 2 in]
                            n1112 = local write "RESULT LAB01-1"(TRUE) -> ()
                            n1113 = local write "DISP LAB01-1"(w2137) -> ()
                          }
                        }
                      }
                      frame False {
                      }
                    }
                  }
                }
              }
              frame #1 {
                # "LAB01-2"
                n1114 = Less?(x=w2140, y=2) -> (x < y?=w2143:bool)
                n1115 = local read "DISP LAB01-2"() -> (w2145:T4)
                n1116 = Unbundle(w2145) -> ("STATUS"=w2146:string)  [unwired: 2 out]
                n1117 = Equal?(x=w2146, y="RUN") -> (x = y?=w2142:bool)
                n1118 = And(x=w2142, y=w2143) -> (x .and. y?=w2141:bool)
                n1119 = case shown="True" w2141 {
                  tunnel: w2145 -> [_ w2151]
                  tunnel: w2140 -> [_ w2155]
                  frame False {
                  }
                  frame True {
                    n1120 = local read "SET LAB01-2"() -> (w2157:T5)
                    n1121 = local read "TDMS LAB01-2"() -> (w2150:refnum<k34>)
                    n1122 = Unbundle(w2157) -> ("CYCLES"=w2148:dbl, "T-RISE mins"=w2154:dbl)  [unwired: 3 out]
                    n1123 = case shown="\"T-RISE TEST\"" w2155 {
                      tunnel: w2154 -> [_ _ w2164]
                      tunnel: [w2159 w2161 w2164] -> w2153
                      tunnel: w2148 -> [w2159 w2161 _]
                      tunnel: ["CHART PASS" "CYCLE PASS" "T-RISE PASS"] -> w2152
                      frame "CHART TEST", Default {
